vi "Write constants.vi"(5 "constants":refnum<class "Constant.lvclass">[](array[class]), 9 "Diagram in":refnum<class "Diagram.lvclass">) -> (3 "Diagram out":refnum<class "Diagram.lvclass">)   [LabVIEW 2014, in "Diagram.lvclass"]
uses:
  Diagram.lvclass
  Constant/Constant.lvclass
  Diagram.lvclass/Diagram.ctl
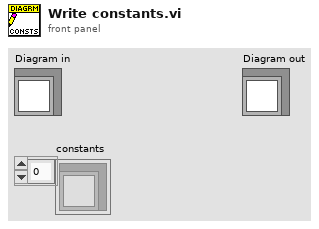
[diagram p1: front panel]
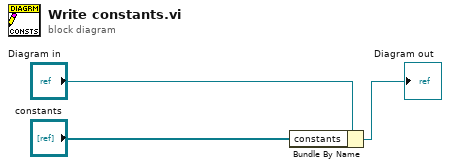
[diagram p0: block diagram]
diagram:
  n1 = Bundle By Name(cluster="Diagram in", "constants"="constants") -> (→"Diagram out":refnum<class "Diagram.lvclass">)
